vi "Configure Reference Levels.vi"(5 "Low Reference (10.0%)":dbl, 7 "Mid Reference (50.0%)":dbl, 8 "error in (no error)":errorcluster, 9 "High Reference (90.0%)":dbl, 10 "Channel (31: All Waveforms)":u16(ring) items=["Channel 1", "Channel 2", "Channel 3", "Channel 4", "Function 1", "Function 2", "Function 3", "Function 4", "Memory 1", "Memory 2", "Memory 3", "Memory 4", "All Waveforms"], 11 "VISA resource name":refnum<visa-resource-name>) -> (0 "error out":errorcluster, 3 "VISA resource name out":refnum<visa-resource-name>)   [LabVIEW 2009, in "Agilent 8000 Series.lvlib"]
doc: "Configures the reference levels in percents for waveform measurements. \n\nYou must call this VI before you call the Read Waveform Measurement.vi or Fetch Waveform Measurement.vi to take a rise time, fall time, width negative, width positive, duty cycle negative, or duty cycle positive measurement."
uses:
  Agilent 8000 Series.lvlib
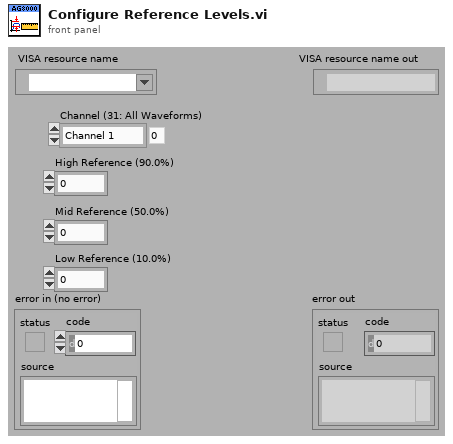
[diagram p1: front panel]
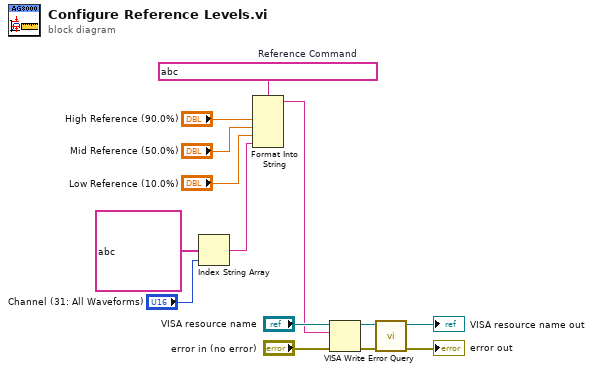
[diagram p0: block diagram]
diagram:
  w8 = string ?  # Reference Command
  n1 = Index String Array(1:"Channel (31: All Waveforms)", 2:string[] ?) -> (0:w1:string)  [unwired: 1 in]
  n2 = Format Into String(format string=w8, "High Reference (90.0%)", "Mid Reference (50.0%)", "Low Reference (10.0%)", w1) -> (resulting string=w4:string)  [unwired: 2 in, 1 out]
  n3 = VISA Write(VISA resource name="VISA resource name", write buffer=w4, error in (no error)="error in (no error)") -> (VISA resource name out=w10:refnum<visa-resource-name>, error out=w9:errorcluster)  [unwired: 1 out]
  n4 = call "Error Query.vi"("error in (no error)"=w9, "VISA resource name"=w10) -> ("error out"=→"error out":errorcluster, "VISA resource name out"=→"VISA resource name out":refnum<visa-resource-name>)  [unwired: 6 in, 2 out]
